vi "Intake Immediate.vi"(8 "Operation":T1, 11 "Intake Power":dbl) -> ()   [LabVIEW 2019]
uses:
  Implementation/Intake Operations.ctl
  Implementation/Intake Setpoints.ctl
  <vilib>/Rock Robotics/WPI/Framework/Completion Status.ctl
  <vilib>/Rock Robotics/WPI/Framework/Completion Notifier.ctl
  <vilib>/Rock Robotics/WPI/Framework/Command Status Info.ctl
panel:
  in  "Description":string
  out "Command Info Out":T2
  in  "Command Info In":T2
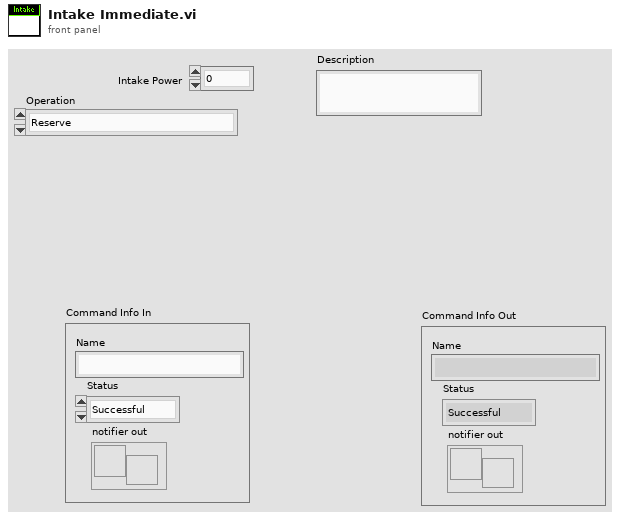
[diagram p1: front panel]
types:
  T1 = typedef "Intake Operations.ctl" = enum16{"Reserve", "Read Current", "Immediate", "Extend", "Retract"}
  T2 = typedef "Command Status Info.ctl" = cluster{"Name":string, "Status":T3, "notifier out":T4}
  T3 = typedef "Completion Status.ctl" = enum16{"Successful", "Aborted", "Incomplete"}
  T4 = typedef "Completion Notifier.ctl" = refnum<notifier>
  T5 = typedef "Intake Setpoints.ctl" = cluster{"Operation":T1, "Intake Power":dbl}
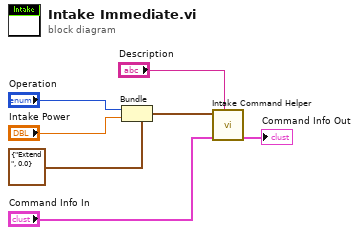
[diagram p0: block diagram]
diagram:
  n1 = Bundle(cluster=T5 {"Operation"=enum."Extend", "Intake Power"=0.0} ("SubSystem Data"), "Operation"="Operation", "Intake Power"="Intake Power") -> (w2:T5)
  n2 = call "Intake Command Helper.vi"("Description"="Description", "Command Info In"="Command Info In", "SubSystem Data"=w2) -> ("Command Info Out"=→"Command Info Out":T2)  [unwired: 6 in, 2 out]
